vi "SensorReadOneLine3times.vi"() -> ()   [LabVIEW 2016]
uses:
  Control/Coordinate.ctl
  Other Models/2010/Status/ControllerDiagPacket.ctl
  Other Models/2010/Status/AxisDiagPacket.ctl
  <vilib>/Instr/_visa.llb/VISA Configure Serial Port (Instr).vi
panel:
  in  "StartPoint 4":T1 {"X" format="%#.5g"; "Y" format="%#.5g"; "Z" format="%#.5g"}
  in  "EndPoint 4":T1 {"X" format="%#.5g"; "Y" format="%#.5g"; "Z" format="%#.6g"}
  in  "StartPoint 3":T1 {"X" format="%#.5g"; "Y" format="%#.5g"; "Z" format="%#.5g"}
  in  "EndPoint 3":T1 {"X" format="%#.5g"; "Y" format="%#.5g"; "Z" format="%#.6g"}
  in  "StartPoint 2":T1 {"X" format="%#.5g"; "Y" format="%#.5g"; "Z" format="%#.5g"}
  in  "EndPoint 2":T1 {"X" format="%#.5g"; "Y" format="%#.5g"; "Z" format="%#.6g"}
  out "Boolean":bool=TRUE
  in  "baud rate":u32=1500000
  in  "data bits":u16=8 min=5 max=8 step=1
  in  "parity":u16(ring)=2 items=["None", "Odd", "Even", "Mark", "Space"]
  in  "stop bits":u16(ring)=10 items=["1"=10, "1.5"=15, "2.0"=20]
  in  "flow control":u16(ring) items=["None"=0, "XON/XOFF"=1, "RTS/CTS"=2, "DTR/DSR"=4]
  in  "VISA resource name":refnum<visa-resource-name>="COM4"
  in  "Speed":dbl format="%#_13g"
  in  "EndPoint":T1 {"X" format="%#.5g"; "Y" format="%#.5g"; "Z" format="%#.6g"}
  in  "StartPoint":T1 {"X" format="%#.5g"; "Y" format="%#.5g"; "Z" format="%#.5g"}
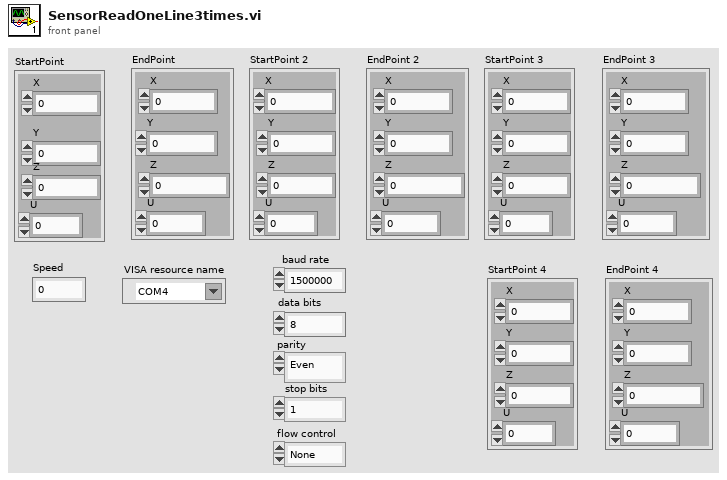
[diagram p1: front panel]
types:
  T1 = typedef "Coordinate.ctl" = cluster{"X":dbl, "Y":dbl, "Z":dbl, "U":dbl}
  T2 = typedef "ControllerDiagPacket.ctl" = cluster{"Number of Diag Packets":i32, "Axes":T3[], "error":errorcluster}
  T3 = typedef "AxisDiagPacket.ctl" = cluster{"Axis Name":string, "Analog Input 0":dbl, "Analog Input 1":dbl, "Axis Fault (num)":i32, "Axis Fault (str)":string, "Axis Fault (bits)":cluster{"AmplifierFault":bool, "AmplifierTemperatureFault":bool, "CcwEndOfTravelLimitFault":bool, "CcwSoftwareLimitFault":bool, "CommunicationLostFault":bool, "CwEndOfTravelLimitFault":bool, "CwSoftwareLimitFault":bool, "EmergencyStopFault":bool, "EncoderFault":bool, "ExternalFault":bool, "FeedbackScalingFault":bool, "GantryMisalignFault ":bool, "HallSensorFault":bool, "InPositionTimeoutFault":bool, "InternalFault":bool, "MarkerSearchFault":bool, "MaxVelocityCommandFault":bool, "MissedInterruptFault":bool, "MotorTemperatureFault":bool, "None":bool, "OverCurrentFault":bool, "PositionErrorFault":bool, "PositionFeedbackFault":bool, "PowerSupplyFault":bool, "ProbeInputFault":bool, "SafeZoneFault":bool, "VelocityErrorFault":bool, "VelocityFeedbackFault":bool, "VoltageClampFault":bool}, "Axis Status (num)":i32, "Axis Status (str)":string, "Axis Status (bits)":cluster{"BacklashActive":bool, "CalibrationEnabled1D":bool, "CalibrationEnabled2D":bool, "CommandValid":bool, "DriveAbortPending":bool, "DrivePending":bool, "Enabling":bool, "GainMappingEnabled":bool, "GantryAligned":bool, "GantryRealigning":bool, "Homed":bool, "Homing":bool, "IFOVEnabled":bool, "JogGenerating":bool, "Jogging":bool, "JoystickControl":bool, "MasterSlaveControl":bool, "MotionBlocked":bool, "MotionClamped":bool, "MoveDone":bool, "None":bool, "NotVirtual":bool, "Profiling":bool, "Stability0":bool, "Stability1":bool, "TrajectoryFiltering":bool, "WaitDone":bool}, "Current Command":sgl, "Current Error":sgl, "Current Feedback":sgl, "Digital Inputs":i32, "Digital Outputs":i32, "Drive Status":i32, "Drive Status (str)":string, "Drive Status (bits)":cluster{"AccelerationPhase":bool, "AutofocusActive":bool, "BrakeOutput":bool, "CcwEndOfTravelLimitInput":bool, "CosineEncoderError":bool, "CurrentClamp":bool, "CwEndOfTravelLimitInput":bool, "DecelerationPhase":bool, "DualLoopActive":bool, "EmergencyStopInput":bool, "Enabled":bool, "EncoderClipping":bool, "GalvoCalibrationEnabled":bool, "GalvoPowerCorrection":bool, "HallAInput":bool, "HallBInput":bool, "HallCInput":bool, "HighResolutionMode":bool, "HomeLimitInput":bool, "InPosition":bool, "InPosition2":bool, "MarkerInput":bool, "MarkerLatch":bool, "MoveActive":bool, "NoMotorSupply":bool, "None":bool, "PowerLimiting":bool, "ProgrammingFlash":bool, "ProgrammingMXH":bool, "PSOHaltLatch":bool, "ServoControl":bool, "SineEncoderError":bool}, "Position Feedback Auxiliary":dbl, "Position Command":dbl, "Position Error":dbl, "Position Feedback":dbl, "Program Position Command":dbl, "Program Position Error":dbl, "Program Position Feedback":dbl, "Velocity Command":dbl, "Velocity Error":dbl, "Velocity Feedback":dbl}
  T4 = cluster{"ControllerDiagPacket":T2, "read buffer":string}
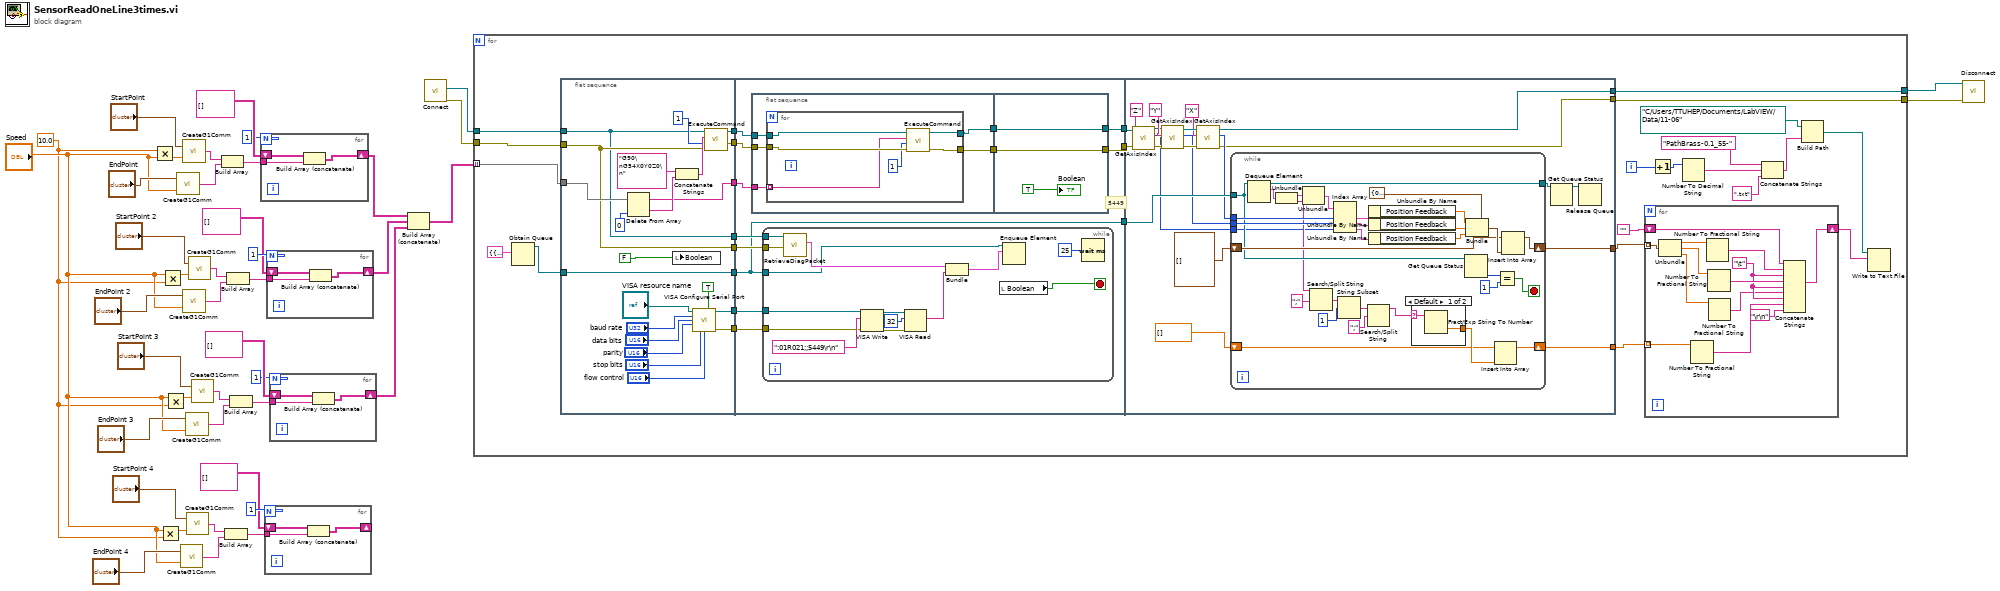
[diagram p0: block diagram]
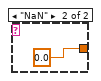
[diagram p2: hidden frame]
diagram:
  w2 = 10.0
  n1 = Multiply(x=w2, y="Speed") -> (x*y=w13:dbl)
  n2 = Multiply(x="Speed", y=w2) -> (x*y=w10:dbl)
  n3 = Multiply(x="Speed", y=w2) -> (x*y=w12:dbl)
  n4 = Multiply(x="Speed", y=w2) -> (x*y=w11:dbl)
  n5 = call "CreateG1Comm.vi"("Numeric"="Speed", "StartPoint"="EndPoint") -> ("String out"=w32:string)
  n6 = call "CreateG1Comm.vi"("Numeric"="Speed", "StartPoint"="EndPoint 4") -> ("String out"=w9:string)
  n7 = call "CreateG1Comm.vi"("Numeric"=w13, "StartPoint"="StartPoint") -> ("String out"=w33:string)
  n8 = call "CreateG1Comm.vi"("Numeric"="Speed", "StartPoint"="EndPoint 2") -> ("String out"=w31:string)
  n9 = call "CreateG1Comm.vi"("Numeric"="Speed", "StartPoint"="EndPoint 3") -> ("String out"=w18:string)
  n10 = call "CreateG1Comm.vi"("Numeric"=w10, "StartPoint"="StartPoint 4") -> ("String out"=w8:string)
  n11 = call "CreateG1Comm.vi"("Numeric"=w12, "StartPoint"="StartPoint 2") -> ("String out"=w30:string)
  n12 = call "CreateG1Comm.vi"("Numeric"=w11, "StartPoint"="StartPoint 3") -> ("String out"=w19:string)
  n13 = Build Array(w33, w32) -> (w38:string[])
  n14 = Build Array(w8, w9) -> (w4:string[])
  n15 = Build Array(w30, w31) -> (w25:string[])
  n16 = Build Array(w19, w18) -> (w24:string[])
  n17 = for {
    N: 1 -> [_]
    tunnel: w38 -> [w45]
    shift-right: [w44] -> w17
    shift-left: string[][] [] -> [w43]
    n18 = Build Array (concatenate)(w43, w45) -> (w44:string[][])
  }
  n19 = for {
    N: 1 -> [_]
    tunnel: w4 -> [w48]
    shift-right: [w47] -> _
    shift-left: string[][] [] -> [w46]
    n20 = Build Array (concatenate)(w46, w48) -> (w47:string[][])
  }
  n21 = for {
    N: 1 -> [_]
    tunnel: w25 -> [w51]
    shift-right: [w50] -> w16
    shift-left: string[][] [] -> [w49]
    n22 = Build Array (concatenate)(w49, w51) -> (w50:string[][])
  }
  n23 = for {
    N: 1 -> [_]
    tunnel: w24 -> [w54]
    shift-right: [w53] -> w15
    shift-left: string[][] [] -> [w52]
    n24 = Build Array (concatenate)(w52, w54) -> (w53:string[][])
  }
  n25 = Build Array (concatenate)(w17, w16, w15) -> (w14:string[][])
  n26 = call "Connect.vi"() -> ("error out"=w42:errorcluster, "controller"=w41:refnum<k24>)  [unwired: 10 in]
  n27 = for {
    tunnel: w14 -> [w73] mode=indexing
    tunnel: w42 -> [w66]
    tunnel: w41 -> [w65]
    tunnel: [w56] -> w40
    tunnel: [w55] -> w39
    i -> [w64]
    # "5449"
    n28 = Obtain Queue(element data type=cluster{"ControllerDiagPacket":T2, string} {"ControllerDiagPacket"={"Number of Diag Packets"=0, "Axes"=[], "error"={"status"=FALSE, "code"=0, "source"=""}}, ""}) -> (queue out=w71:refnum<queue>)  [unwired: 4 in, 2 out]
    n29 = flat-sequence {
      tunnel: [w113] -> w84
      tunnel: [w117] -> w83
      tunnel: [w118] -> w82
      tunnel: w73 -> [w119]
      tunnel: [w98] -> w81
      tunnel: [w99] -> w80
      tunnel: w71 -> [w111]
      tunnel: [w111] -> w79
      tunnel: [w103] -> w78
      tunnel: [w102] -> w77
      tunnel: w66 -> [w99]
      tunnel: w65 -> [w98]
      tunnel: [w126] -> w76
      tunnel: w84 -> [w120]
      tunnel: w83 -> [w122]
      tunnel: w82 -> [w121]
      tunnel: w81 -> [w130]
      tunnel: w80 -> [w131]
      tunnel: w79 -> [w129]
      tunnel: [w129] -> w75
      tunnel: w78 -> [w128]
      tunnel: w77 -> [w127]
      tunnel: [w123] -> w74
      tunnel: w76 -> [w167]
      tunnel: w75 -> [w180]
      tunnel: [w169] -> w67
      tunnel: [w168] -> w68
      tunnel: w74 -> [w166]
      tunnel: [w161] -> w56
      tunnel: [w160] -> w55
      frame #0 {
        n30 = Delete From Array(array=w119, index=0) -> (deleted portion=w114:string, array with subset deleted=w113:string[])  [unwired: 1 in]
        n31 = local write "Boolean"(FALSE) -> ()
        n32 = Concatenate Strings("G90\nG54X0Y0Z0\n", w114) -> (w112:string)
        n33 = call-poly "VISA Configure Serial Port"("VISA resource name"="VISA resource name", "Enable Termination\nChar (T)"=TRUE, "baud rate (9600)"="baud rate", "data bits (8)"="data bits", "parity (0:none)"="parity", "stop bits (10: 1 bit)"="stop bits", "flow control (0:none)"="flow control") -> ("VISA resource name out"=w103:refnum<visa-resource-name>, "error out"=w102:errorcluster)  [unwired: 7 in]
        n34 = call "ExecuteCommand.vi"("error in (no error)"=w99, "taskId"=1, "Command Code"=w112, "controller in"=w98) -> ("error out"=w118:errorcluster, "controller out"=w117:refnum<k24>)  [unwired: 5 in, 1 out]
      }
      frame #1 {
        n35 = flat-sequence {
          tunnel: [w136] -> w125
          tunnel: [w135] -> w124
          tunnel: w122 -> [w134]
          tunnel: w121 -> [w133]
          tunnel: w120 -> [w132]
          tunnel: [w144] -> w126
          tunnel: w125 -> [w144]
          tunnel: w124 -> [w143]
          tunnel: [w143] -> w123
          frame #0 {
            n36 = for {
              tunnel: w132 -> [w140] mode=indexing
              tunnel: w134 -> [w141]
              tunnel: w133 -> [w142]
              tunnel: [w138] -> w136
              tunnel: [w137] -> w135
              n37 = call "ExecuteCommand.vi"("error in (no error)"=w142, "taskId"=1, "Command Code"=w140, "controller in"=w141) -> ("error out"=w138:errorcluster, "controller out"=w137:refnum<k24>)  [unwired: 5 in, 1 out]
            }
          }
          frame #1 {
            "Boolean" <- TRUE
          }
        }
        n38 = while {
          tunnel: w130 -> [w159]
          tunnel: w131 -> [w158]
          tunnel: w129 -> [w146]
          tunnel: w128 -> [w155]
          tunnel: w127 -> [w153]
          stop <- w147 stop-if-true
          n39 = call "RetrieveDiagPacket.vi"("error in (no error)"=w158, "Controller In"=w159) -> ("ControllerDiagPacket"=w150:T2)  [unwired: 7 in, 2 out]
          n40 = VISA Write(VISA resource name=w155, write buffer=":01R021;;5449\r\n", error in (no error)=w153) -> (VISA resource name out=w156:refnum<visa-resource-name>, error out=w152:errorcluster)  [unwired: 1 out]
          n41 = VISA Read(VISA resource name=w156, byte count=u32 32, error in (no error)=w152) -> (read buffer=w149:string)  [unwired: 3 out]
          n42 = Bundle("ControllerDiagPacket"=w150, "read buffer"=w149) -> (w148:T4)  [unwired: 1 in]
          n43 = local read "Boolean"() -> (w147:bool)
          n44 = Enqueue Element(queue=w146, element=w148) -> ()  [unwired: 2 in, 3 out]
          n45 = Wait (ms)(milliseconds to wait=25) -> ()  [unwired: 1 out]
        }
      }
      frame #2 {
        n46 = call "GetAxisIndex.vi"("error in (no error)"=w167, "axis name"="Z", "controller in"=w166) -> ("error out"=w164:errorcluster, "axis index"=w162:i32, "controller out"=w165:refnum<k24>)  [unwired: 6 in]
        n47 = call "GetAxisIndex.vi"("error in (no error)"=w164, "axis name"="Y", "controller in"=w165) -> ("error out"=w178:errorcluster, "axis index"=w174:i32, "controller out"=w179:refnum<k24>)  [unwired: 6 in]
        n48 = call "GetAxisIndex.vi"("error in (no error)"=w178, "axis name"="X", "controller in"=w179) -> ("error out"=w160:errorcluster, "axis index"=w175:i32, "controller out"=w161:refnum<k24>)  [unwired: 6 in]
        n49 = while {
          tunnel: w175 -> [w210]
          tunnel: w174 -> [w209]
          shift-right: [w202] -> w168
          shift-left: cluster{"X":dbl, "Y":dbl, "Y 2":dbl}[] [] -> [w200]
          tunnel: [w201] -> w172
          tunnel: w180 -> [w196]
          shift-right: [w184] -> w169
          shift-left: dbl[] [] -> [w185]
          tunnel: w162 -> [w183]
          stop <- w198 stop-if-true
          n50 = Dequeue Element(queue=w196) -> (queue out=w201:refnum<queue>, element=w195:cluster{"ControllerDiagPacket":T2, string})  [unwired: 2 in, 2 out]
          n51 = Unbundle(w195) -> ("ControllerDiagPacket"=w194:T2, w188:string)
          n52 = Unbundle(w194) -> ("Axes"=w211:T3[])  [unwired: 2 out]
          n53 = Search/Split String(string=w188, search string/char (-)=";") -> (match + rest of string=w189:string)  [unwired: 1 in, 2 out]
          n54 = Index Array(array=w211, index #1=w210, index #2=w209, index #3=w183) -> (element #1=w208:T3, element #2=w207:T3, element #3=w182:T3)
          n55 = String Subset(string=w189, offset (0)=1) -> (substring=w191:string)  [unwired: 1 in]
          n56 = Search/Split String(string=w191, search string/char (-)=";") -> (substring before match=w187:string)  [unwired: 1 in, 2 out]
          n57 = Unbundle By Name(w208) -> ("Position Feedback"=w205:dbl)
          n58 = Unbundle By Name(w207) -> ("Position Feedback"=w204:dbl)
          n59 = Unbundle By Name(w182) -> ("Position Feedback"=w181:dbl)
          n60 = case shown="Default" w187 {
            selector: w187 -> [w213 _]
            tunnel: [w212 0.0] -> w186
            frame Default {
              n61 = Fract/Exp String To Number(string=w213) -> (number=w212:dbl)  [unwired: 3 in, 1 out]
            }
            frame "NaN" {
            }
          }
          n62 = Get Queue Status(queue=w196) -> (# elements in queue=w199:i32)  [unwired: 2 in, 7 out]
          n63 = Bundle(cluster=cluster{"X":dbl, "Y":dbl, "Z":dbl} {"X"=0.0, "Y"=0.0, "Z"=0.0}, "X"=w205, "Y"=w204, "Z"=w181) -> (w203:cluster{"X":dbl, "Y":dbl, "Z":dbl})
          n64 = Insert Into Array(array=w185, new element=w186) -> (w184:dbl[])  [unwired: 1 in]
          n65 = Equal?(x=w199, y=1) -> (x = y?=w198:bool)
          n66 = Insert Into Array(array=w200, new element=w203) -> (w202:cluster{"X":dbl, "Y":dbl, "Y 2":dbl}[])  [unwired: 1 in]
        }
        n67 = Get Queue Status(queue=w172) -> (queue out=w171:refnum<queue>)  [unwired: 2 in, 7 out]
        n68 = Release Queue(queue=w171) -> ()  [unwired: 2 in, 3 out]
      }
    }
    n69 = for {
      tunnel: w68 -> [w97] mode=indexing
      tunnel: w67 -> [w94] mode=indexing
      shift-right: [w90] -> w70
      shift-left: "" -> [w91]
      w89 = "\t"
      n70 = Unbundle(w97) -> ("X"=w96:dbl, "Y"=w95:dbl, "Y 2"=w88:dbl)
      n71 = Number To Fractional String(number=w94) -> (F-format string=w86:string)  [unwired: 3 in]
      n72 = Number To Fractional String(number=w96) -> (F-format string=w93:string)  [unwired: 3 in]
      n73 = Number To Fractional String(number=w95) -> (F-format string=w92:string)  [unwired: 3 in]
      n74 = Number To Fractional String(number=w88) -> (F-format string=w87:string)  [unwired: 3 in]
      n75 = Concatenate Strings(w91, w93, w89, w92, w89, w87, w89, w86, "\r\n") -> (w90:string)
    }
    n76 = Increment(x=w64) -> (x+1=w59:i32)
    n77 = Number To Decimal String(number=w59) -> (decimal integer string=w63:string)  [unwired: 1 in]
    n78 = Concatenate Strings("PathBrass-0.1_55-", w63, ".txt") -> (w61:string)
    n79 = Build Path(base path=path "C:/Users/TTUHEP/Documents/LabVIEW/Data/11-06" ("file (use dialog) 2"), name or relative path=w61) -> (appended path=w60:path)
    n80 = Write to Text File(file (use dialog)=w60, text=w70) -> ()  [unwired: 2 in, 3 out]
  }
  n81 = call "Disconnect.vi"("error in (no error)"=w39, "controller"=w40) -> ()  [unwired: 9 in, 1 out]
